vi "To JSON String.vi"(8 "error in (no error)":errorcluster, 11 "id in":refnum<class "id.lvclass">) -> (0 "error out":errorcluster, 2 "JSON String":string, 3 "id out":refnum<class "id.lvclass">)   [LabVIEW 2016, in "id.lvclass"]
uses:
  id.lvclass
  <vilib>/NI/JSON Support for LabVIEW/JSON Data Classes/JSON Datatype/JSON Null.lvclass
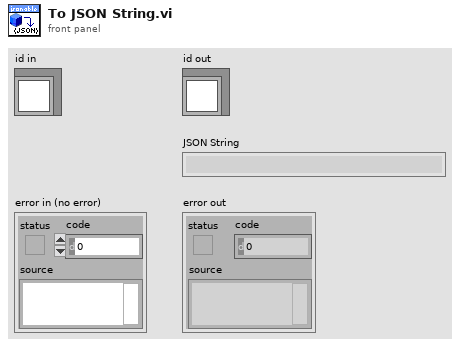
[diagram p1: front panel]
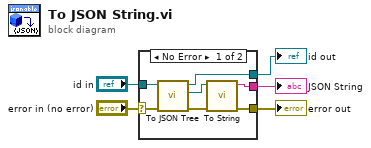
[diagram p0: block diagram]
diagram:
  n1 = case shown="No Error" "error in (no error)" {
    selector: "error in (no error)" -> [w11 w14]
    tunnel: [w7 w14] -> w4
    tunnel: [w10 w13] -> w2
    tunnel: "id in" -> [w12 w13]
    tunnel: [w8 _] -> w1
    frame No Error {
      n2 = call "To JSON Tree.vi"("error in (no error)"=w11, "id in"=w12) -> ("error out"=w6:errorcluster, "JSON out"=w9:refnum<class "JSON Null.lvclass">, "id out"=w10:refnum<class "id.lvclass">)  [unwired: 7 in]
      n3 = call-dynamic "To String.vi"("error in (no error)"=w6, "JSON Datatype in"=w9) -> ("error out"=w7:errorcluster, "String"=w8:string)  [unwired: 8 in]
    }
    frame Error {
    }
  }
  "error out" <- w4
  "id out" <- w2
  "JSON String" <- w1
